vi "Firmware Independent FPGA Interface Example.vi"() -> ()   [LabVIEW 2010]
uses:
  <vilib>/userDefined/High Color/nirio_resource_hc.ctl
  Firmware Independent PID Interface/TypeDefs/ControlI16.ctl
  Firmware Independent PID Interface/TypeDefs/IndicatorU32.ctl
  Firmware Independent PID Interface/Firmware Independent PID Interface.lvclass
  Firmware Independent PID Interface/FPGA Read - U32.vi
  Firmware Independent PID Interface/FPGA Write - I16.vi
panel:
  in  "Run FPGA":bool
  in  "Setpoints":dbl[](array[numeric])
  in  "RIO Resource":T1="RIO0"
  out "Loop Rate":dbl format="%#_6p"
  in  "Bitfile Path":path
  in  "Stop":bool
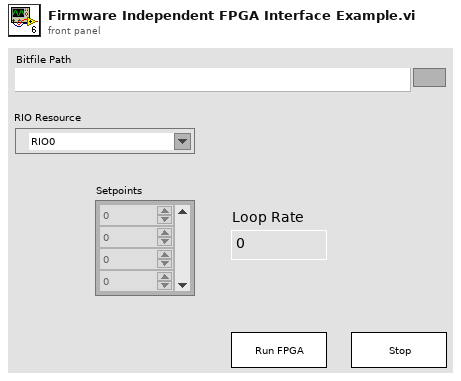
[diagram p1: front panel]
types:
  T1 = typedef "nirio_resource_hc.ctl" = tag
  T2 = typedef "Firmware Independent PID Interface.lvclass/IndicatorU32.ctl" = enum16{"PID.Num Ticks"}
  T3 = typedef "Firmware Independent PID Interface.lvclass/ControlI16.ctl" = enum16{"PID.Setpoint.PID 0", "PID.Setpoint.PID 2", "PID.Proportional Gain.PID 2", "PID.Integral Gain.PID 2", "PID.Derivative Gain.PID 2", "PID.Setpoint.PID 3", "PID.Proportional Gain.PID 3", "PID.Integral Gain.PID 3", "PID.Derivative Gain.PID 3", "PID.Setpoint.PID 1", "PID.Proportional Gain.PID 1", "PID.Integral Gain.PID 1", "PID.Derivative Gain.PID 1", "PID.Proportional Gain.PID 0", "PID.Integral Gain.PID 0", "PID.Derivative Gain.PID 0"}
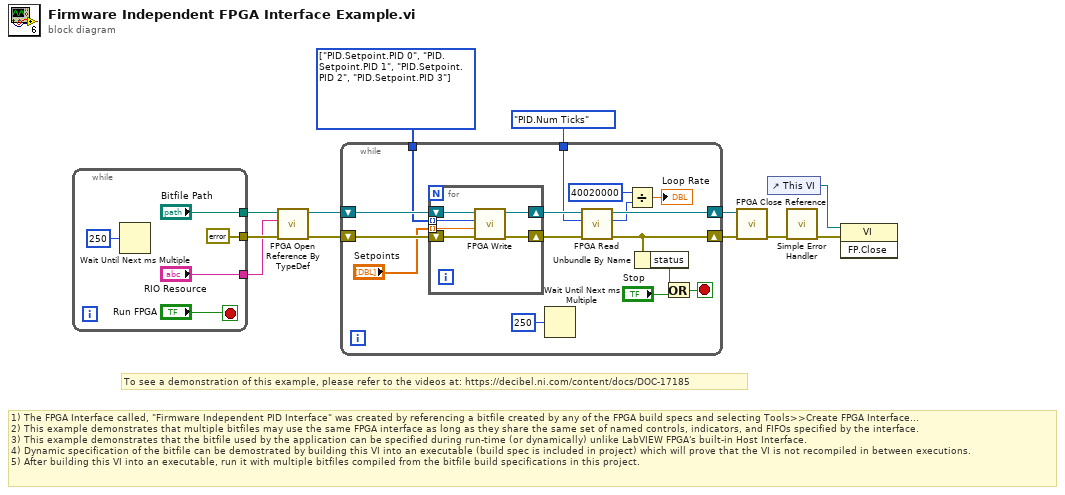
[diagram p0: block diagram]
diagram:
  w10 = T3[] [enum."PID.Setpoint.PID 0", enum."PID.Setpoint.PID 1", enum."PID.Setpoint.PID 2", enum."PID.Setpoint.PID 3"] items=["PID.Setpoint.PID 0", "PID.Setpoint.PID 2", "PID.Proportional Gain.PID 2", "PID.Integral Gain.PID 2", "PID.Derivative Gain.PID 2", "PID.Setpoint.PID 3", "PID.Proportional Gain.PID 3", "PID.Integral Gain.PID 3", "PID.Derivative Gain.PID 3", "PID.Setpoint.PID 1", "PID.Proportional Gain.PID 1", "PID.Integral Gain.PID 1", "PID.Derivative Gain.PID 1", "PID.Proportional Gain.PID 0", "PID.Integral Gain.PID 0", "PID.Derivative Gain.PID 0"]
  # "1) The FPGA Interface called, \"Firmware Independent PID Interface\" was created by referencing a bitfile created by any of the FPGA build specs and selecting Tools>>Create FPGA Interface...\n2) This example demonstrates that multiple bitfiles may use the same FPGA interface as long as they share the same set of named controls, indicators, and FIFOs specified by the interface.\n3) This example demonstrates that the bitfile used by the application can be specified during run-time (or dynamically) unlike LabVIEW FPGA's built-in Host Interface.\n4) Dynamic specification of the bitfile can be demostrated by building this VI into an executable (build spec is included in project) which will prove that the VI is not recompiled in between executions.\n5) After building this VI into an executable, run it with multiple bitfiles compiled from the bitfile build specifications in this project."
  # "To see a demonstration of this example, please refer to the videos at: https://decibel.ni.com/content/docs/DOC-17185"
  n1 = while {
    tunnel: [errorcluster {"status"=FALSE, "code"=0, "source"=""} ("error in (no error)")] -> w5
    tunnel: ["RIO Resource"] -> w4
    tunnel: ["Bitfile Path"] -> w3
    stop <- "Run FPGA" stop-if-true
    n2 = Wait Until Next ms Multiple(millisecond multiple=u32 250) -> ()  [unwired: 1 out]
  }
  n3 = call "FPGA Open Reference By TypeDef.vi"("error in (no error)"=w5, "FPGA Resource"=w4, "Bitfile Path"=w3) -> ("error out"=w11:errorcluster, "FPGA Session"=w12:refnum<class "Firmware Independent PID Interface.lvclass">)  [unwired: 7 in]
  n4 = while {
    tunnel: w10 -> [w31]
    shift-right: [w28] -> w9
    shift-left: w12 -> [w33]
    tunnel: IndicatorU32."PID.Num Ticks" ("Indicator") -> [w29]
    shift-right: [w22] -> w7
    shift-left: w11 -> [w32]
    stop <- w24 stop-if-true
    n5 = for {
      tunnel: w31 -> [w37] mode=indexing
      shift-right: [w36] -> w21
      shift-left: w32 -> [w38]
      shift-right: [w35] -> w30
      shift-left: w33 -> [w39]
      tunnel: "Setpoints" -> [w34] mode=indexing
      n6 = call-poly "FPGA Write.vi"("error in (no error)"=w38, "Value"=w34, "Control"=w37, "FPGA Session In"=w39) -> ("error out"=w36:errorcluster, "FPGA Session Out"=w35:refnum<class "Firmware Independent PID Interface.lvclass">)  [unwired: 6 in]
    }
    n7 = Wait Until Next ms Multiple(millisecond multiple=u32 250) -> ()  [unwired: 1 out]
    n8 = call-poly "FPGA Read.vi"("error in (no error)"=w21, "Indicator"=w29, "FPGA Session In"=w30) -> ("error out"=w22:errorcluster, "Value"=w26:u32, "FPGA Session Out"=w28:refnum<class "Firmware Independent PID Interface.lvclass">)  [unwired: 6 in]
    n9 = Divide(x=40020000, y=w26) -> (x/y=→"Loop Rate":dbl)
    n10 = Unbundle By Name(w22) -> ("status"=w18:bool)
    n11 = Or(x=w18, y="Stop") -> (x .or. y?=w24:bool)
  }
  n12 = call-dynamic "FPGA Close Reference.vi"("error in (no error)"=w7, "FPGA Session In"=w9) -> ("error out"=w6:errorcluster)  [unwired: 9 in]
  n13 = control-ref of="This VI"() -> (w1:refnum<vi>)
  n14 = call <vilib>:"Simple Error Handler.vi"("error in (no error)"=w6) -> ("error out"=w2:errorcluster)  [unwired: 4 in, 4 out]
  n15 = invoke class="VI" method="FP.Close"(reference=w1, error in=w2) -> ()  [unwired: 1 in, 3 out]
